vi "_test.vi"() -> ()   [LabVIEW 2019]
uses:
  _support/fpMgr/fpMgr.lvclass
panel:
  out "Matched":bool
  out "error out":errorcluster
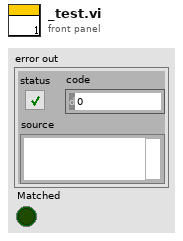
[diagram p1: front panel]
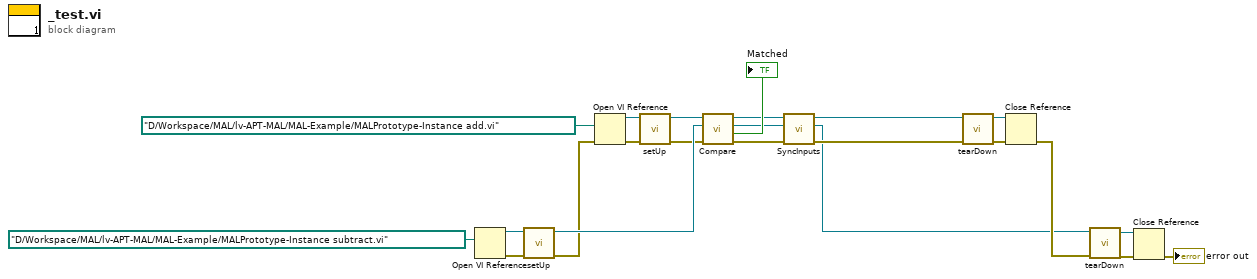
[diagram p0: block diagram]
diagram:
  n1 = Open VI Reference(vi path=path "D:/Workspace/MAL/lv-APT-MAL/MAL-Example/MALPrototype-Instance subtract.vi") -> (vi reference=w19:refnum<vi>, error out=w18:errorcluster)  [unwired: 5 in]
  n2 = call "setUp.vi"("error in (no error)"=w18, "VI in"=w19) -> ("error out"=w15:errorcluster, "fpMgr out"=w16:refnum<class "fpMgr.lvclass">)  [unwired: 8 in]
  n3 = Open VI Reference(vi path=path "D:/Workspace/MAL/lv-APT-MAL/MAL-Example/MALPrototype-Instance add.vi", error in (no error)=w15) -> (vi reference=w21:refnum<vi>, error out=w20:errorcluster)  [unwired: 4 in]
  n4 = call "setUp.vi"("error in (no error)"=w20, "VI in"=w21) -> ("error out"=w14:errorcluster, "fpMgr out"=w17:refnum<class "fpMgr.lvclass">)  [unwired: 8 in]
  n5 = call "Compare.vi"("error in (no error)"=w14, "fpMgr in"=w16, "Shell in"=w17) -> ("error out"=w5:errorcluster, "Matched"=→"Matched":bool, "fpMgr out"=w2:refnum<class "fpMgr.lvclass">, "Shell out"=w6:refnum<class "fpMgr.lvclass">)  [unwired: 5 in]
  n6 = call "SyncInputs.vi"("error in (no error)"=w5, "fpMgr in"=w2, "Shell in"=w6) -> ("error out"=w4:errorcluster, "fpMgr out"=w1:refnum<class "fpMgr.lvclass">, "Shell out"=w3:refnum<class "fpMgr.lvclass">)  [unwired: 6 in]
  n7 = call "tearDown.vi"("error in (no error)"=w4, "fpMgr in"=w3) -> ("error out"=w12:errorcluster, "VI"=w13:refnum<vi>)  [unwired: 8 in]
  n8 = Close Reference(reference=w13, error in (no error)=w12) -> (error out=w11:errorcluster)
  n9 = call "tearDown.vi"("error in (no error)"=w11, "fpMgr in"=w1) -> ("error out"=w9:errorcluster, "VI"=w10:refnum<vi>)  [unwired: 8 in]
  n10 = Close Reference(reference=w10, error in (no error)=w9) -> (error out=→"error out":errorcluster)
